vi "DriveModuleControl.vi"(8 "error in":errorcluster, 9 "Actual State":T1={"Speed"=0.0, "Angle"={"VALUE"=0.0, "COS"=1.0, "SIN"=0.0}} {"Angle"."SIN" format="%13.4f"; "Angle"."COS" format="%13.4f"; "Angle"."VALUE" format="%13.4f"}, 10 "Desired State":T1={"Speed"=0.0, "Angle"={"VALUE"=0.0, "COS"=1.0, "SIN"=0.0}} {"Angle"."SIN" format="%13.4f"; "Angle"."COS" format="%13.4f"; "Angle"."VALUE" format="%13.4f"}, 11 "ModualNamePrefix":i32) -> (0 "error out":errorcluster)   [LabVIEW 2023]
uses:
  <vilib>/Rock Robotics/WPI/ThirdParty/JAS_Junk/TrajLib/TypeDef/SWERVE_DRIVE_MODULE_STATE.ctl
  <vilib>/Rock Robotics/WPI/ThirdParty/JAS_Junk/TrajLib/TypeDef/ROTATION2D.ctl
  <vilib>/Rock Robotics/WPI/ThirdParty/JAS_Junk/TrajLib/Rotation2d_Minus.vi
  <vilib>/Rock Robotics/WPI/ThirdParty/JAS_Junk/TrajLib/Rotation2d_GetRadians.vi
  <vilib>/Rock Robotics/WPI/ThirdParty/JAS_Junk/TrajLib/SwerveModuleState_New.vi
  <vilib>/Rock Robotics/WPI/ThirdParty/JAS_Junk/TrajLib/Rotation2d_RotateBy.vi
  <vilib>/Rock Robotics/WPI/ThirdParty/JAS_Junk/TrajLib/Rotation2d_CreateAngle.vi
  <vilib>/Rock Robotics/WPI/ThirdParty/JAS_Junk/TrajLib/SimpleMotorFF_Calculate.vi
  <vilib>/Rock Robotics/WPI/ThirdParty/JAS_Junk/TrajLib/PIDController_AtSetpoint.vi
  <vilib>/Rock Robotics/WPI/ThirdParty/JAS_Junk/TrajLib/PIDController_SetPIDF.vi
  <vilib>/Rock Robotics/WPI/ThirdParty/JAS_Junk/TrajLib/PIDController_SetDerivativeFilter.vi
  <vilib>/Rock Robotics/WPI/ThirdParty/JAS_Junk/TrajLib/PIDController_SetIntegratorRange.vi
  <vilib>/Rock Robotics/WPI/ThirdParty/JAS_Junk/TrajLib/PIDController_SetTolerancePandV.vi
  <vilib>/Rock Robotics/WPI/ThirdParty/JAS_Junk/TrajLib/PIDController_DisableContinousInput.vi
  <vilib>/Rock Robotics/WPI/ThirdParty/JAS_Junk/TrajLib/PIDController_EnableContinousInput.vi
  <vilib>/Rock Robotics/WPI/ThirdParty/JAS_Junk/TrajLib/PIDController_Reset.vi
  <vilib>/Rock Robotics/WPI/ThirdParty/JAS_Junk/TrajLib/PIDController_New.vi
  <vilib>/Rock Robotics/WPI/ThirdParty/JAS_Junk/TrajLib/PIDController_SetOutputLimits.vi
  <vilib>/Rock Robotics/WPI/ThirdParty/JAS_Junk/TrajLib/VI/PIDController_SetIntegratorZone.vi
  <vilib>/Rock Robotics/WPI/ThirdParty/JAS_Junk/TrajLib/SlewRateLimiter_New.vi
  <vilib>/Rock Robotics/WPI/ThirdParty/JAS_Junk/TrajLib/SlewRateLimiter_Reset.vi
  <vilib>/Rock Robotics/WPI/ThirdParty/JAS_Junk/TrajLib/SlewRateLimiter_Calculate.vi
  <vilib>/Rock Robotics/WPI/ThirdParty/JAS_Junk/TrajLib/SlewRateLimiter_SetRate.vi
  <vilib>/Rock Robotics/WPI/ThirdParty/JAS_Junk/TrajLib/Rotation2d_UnaryMinus.vi
  <vilib>/Rock Robotics/WPI/ThirdParty/JAS_Junk/TrajLib/Rotation2d_CreateXY.vi
  <vilib>/Rock Robotics/WPI/ThirdParty/JAS_Junk/TrajLib/PIDController_NewPeriod.vi
  <vilib>/Rock Robotics/WPI/ThirdParty/JAS_Junk/TrajLib/Util_GetTime.vi
  <vilib>/Rock Robotics/WPI/ThirdParty/JAS_Junk/TrajLib/Util_CalcDist.vi
  <vilib>/Rock Robotics/SystemInterfaces/NetworkCommunication/NetComm_UsageReport_report.vi
  <vilib>/Rock Robotics/WPI/ThirdParty/JAS_Junk/TrajLib/VI/Util_GetTime_U32.vi
  DriveGlobal.vi
  <vilib>/Rock Robotics/SystemInterfaces/Utilities/FPGA_UtilitiesRead LocalTime.vi
  <vilib>/Rock Robotics/WPI/ThirdParty/JAS_Junk/TrajLib/VI/Util_GetTime_U64.vi
  <vilib>/Rock Robotics/WPI/ThirdParty/Phoenix-LabVIEW/CANCoder/CTRE_Phoenix_CANcoder_RefNumRegistryGet.vi
  <vilib>/Rock Robotics/WPI/MotorControl/WPI_MotorControlRefNum Registry Get.vi
  <vilib>/Rock Robotics/Network Tables/NT Write Number.vi
  <vilib>/Rock Robotics/WPI/ThirdParty/JAS_Junk/TrajLib/Globals/Util_LibraryGlobals.vi
  <vilib>/Rock Robotics/WPI/ThirdParty/JAS_Junk/TrajLib/PIDController_AdvCalculate_FF_Sp_Pv.vi
  <vilib>/Rock Robotics/WPI/ThirdParty/JAS_Junk/TrajLib/Trajectory_Library.lvlib
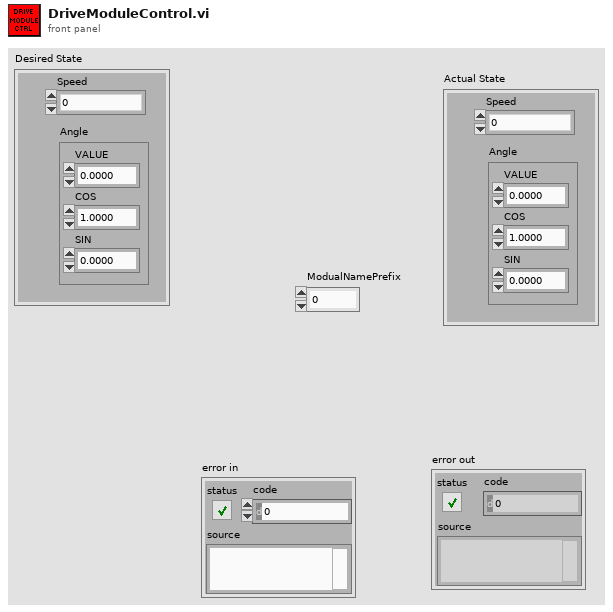
[diagram p1: front panel]
types:
  T1 = typedef "Trajectory_Library.lvlib/SWERVE_DRIVE_MODULE_STATE.ctl" = cluster{"Speed":dbl, "Angle":T2}
  T2 = typedef "Trajectory_Library.lvlib/ROTATION2D.ctl" = cluster{"VALUE":dbl, "COS":dbl, "SIN":dbl}
  T3 = typedef "WPI_MotorControlDeviceRef.ctl" = cluster{"DeviceStatus":errorcluster, "Type":T4, "PWM":cluster{"PWM Channel":T5, "DeadBand":T6}, "CAN":cluster{"Device Number":u8, "SetOutput VI Ref":variant, "GetOutput VI Ref":variant, "Enable VI Ref":variant, "Disable VI Ref":variant, "Data":variant}, "Invert":bool, "DIO PWM":cluster{"PWM \"Enable\" Channel":T5, "DIOChannel":T7, "PWM Rate":dbl}}
  T4 = typedef "WPI_MotorControlType.ctl" = enum16{"PWM", "CAN", "DIO PWM"}
  T5 = typedef "FPGA_DIOPWMChannel.ctl" = enum8{"PWM 0", "PWM 1", "PWM 2", "PWM 3", "PWM 4", "PWM 5", "PWM 6", "PWM 7", "PWM 8", "PWM 9", "PWM MXP 0", "PWM MXP 1", "PWM MXP 2", "PWM MXP 3", "PWM MXP 4", "PWM MXP 5", "PWM MXP 6", "PWM MXP 7", "PWM MXP 8", "PWM MXP 9", "Invalid"}
  T6 = typedef "WPI_PWMDeadband.ctl" = cluster{"Name":string, "maxPositivePwm":i32, "minPositivePwm":i32, "centerPwm":i32, "maxNegativePwm":i32, "minNegativePwm":i32, "angularRange":u16}
  T7 = typedef "FPGA_DIOChannel.ctl" = enum8{"DIO 0", "DIO 1", "DIO 2", "DIO 3", "DIO 4", "DIO 5", "DIO 6", "DIO 7", "DIO 8", "DIO 9", "DIO MXP 0", "DIO MXP 1", "DIO MXP 2", "DIO MXP 3", "DIO MXP 4", "DIO MXP 5", "DIO MXP 6", "DIO MXP 7", "DIO MXP 8", "DIO MXP 9", "DIO MXP 10", "DIO MXP 11", "DIO MXP 12", "DIO MXP 13", "DIO MXP 14", "DIO MXP 15", "SPI Port CS1", "SPI Port CS2", "SPI Port CS3", "SPI Port MISO", "SPI Port MOSI", "Invalid"}
  T8 = typedef "Trajectory_Library.lvlib/SIMPLE_MOTOR_FF.ctl" = cluster{"Ks":dbl, "Kv":dbl, "Ka":dbl, "KnInv":dbl}
  T9 = typedef "Trajectory_Library.lvlib/PID_ADV_LIMITS.ctl" = cluster{"MaxInput":dbl, "MinInput":dbl, "Continuous":bool, "MaxOutput":dbl, "MinOutput":dbl}
  T10 = typedef "Trajectory_Library.lvlib/PID_ADV_TUNING.ctl" = cluster{"Kf":dbl, "Kp":dbl, "Ki":dbl, "Kd":dbl, "MaximumIntegral":dbl, "MinimumIntegral":dbl, "Filter Derivative":bool, "IntegralZone":dbl}
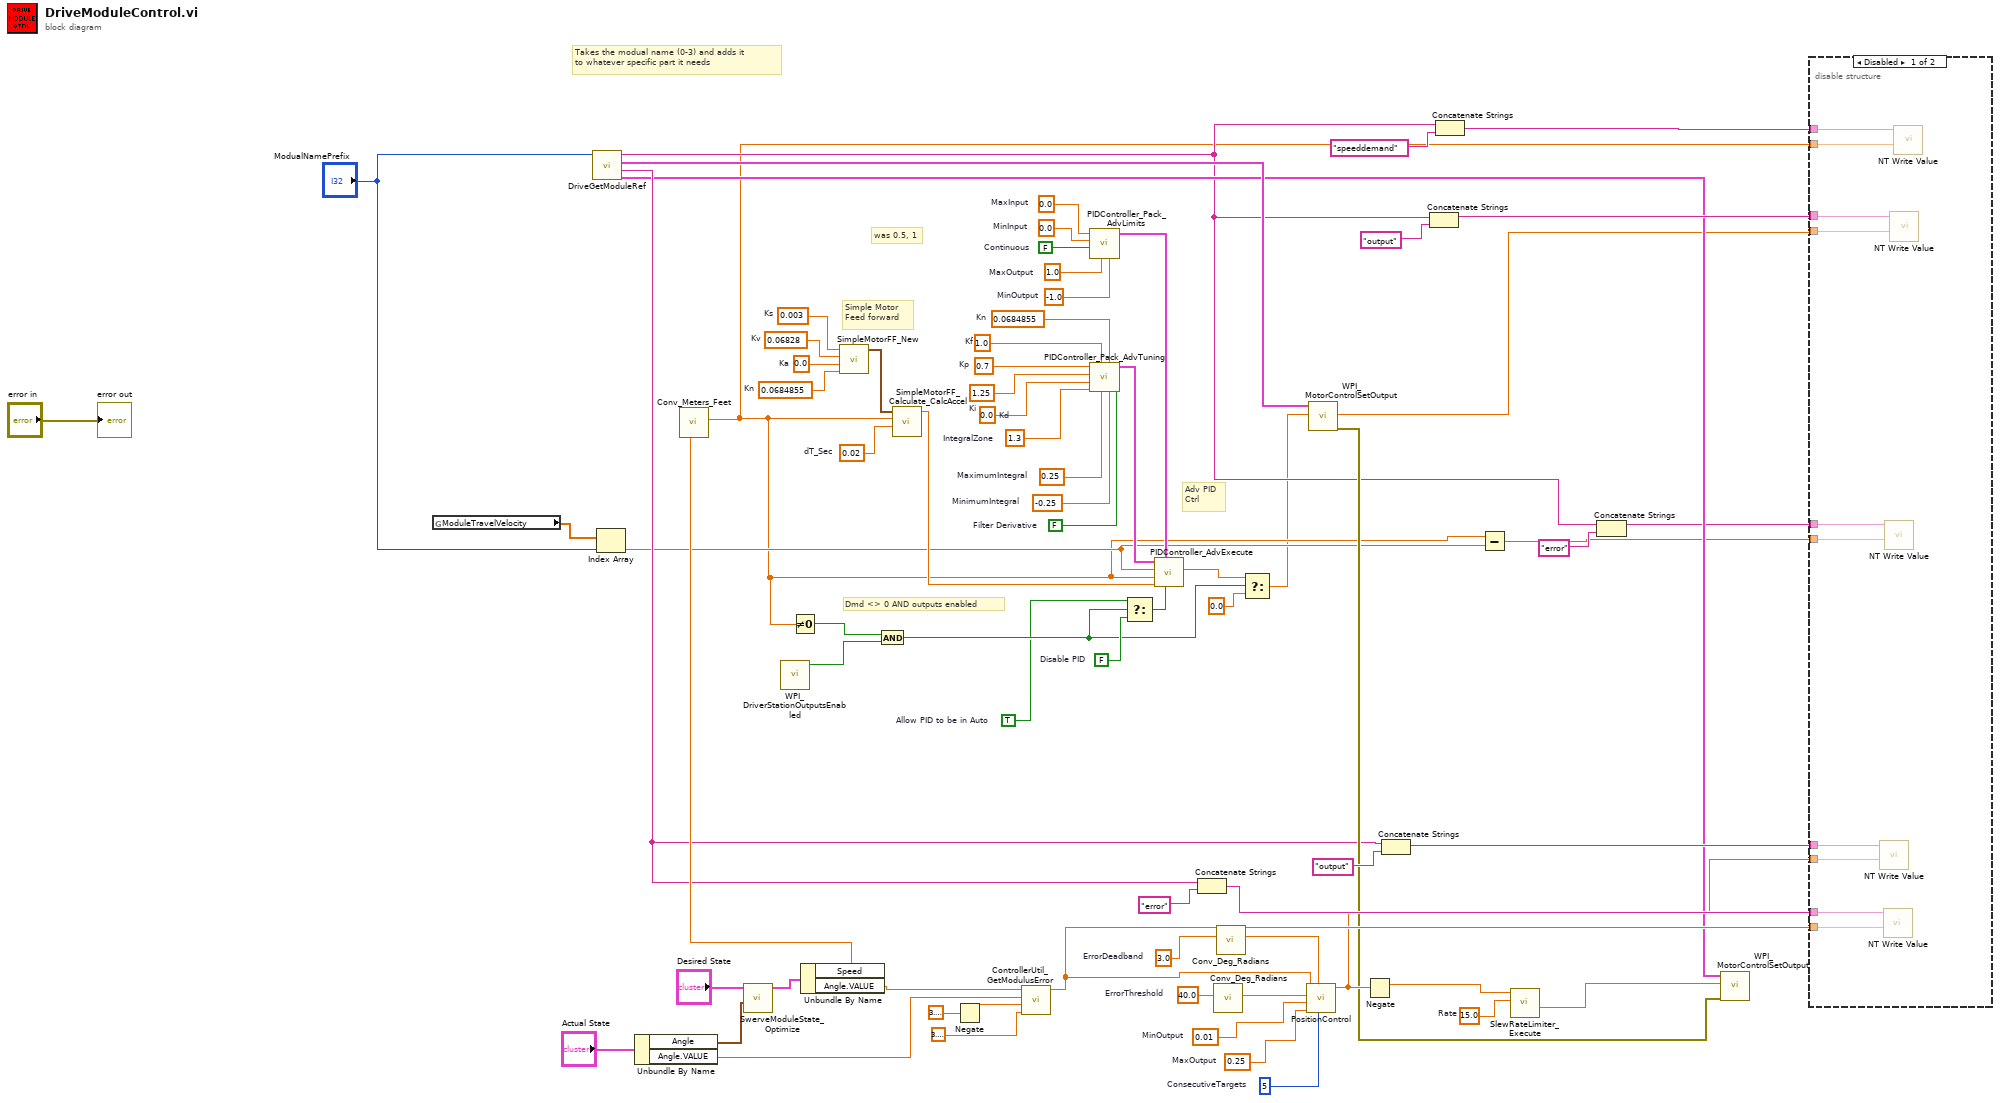
[diagram p0: block diagram]
diagram:
  w1 = 1.3  # IntegralZone
  w4 = 15.0  # Rate
  w5 = TRUE  # Allow PID to be in Auto
  w7 = FALSE  # Disable PID
  w20 = 0.0684855  # Kn
  w37 = 0.7  # Kp
  w36 = 1.25  # Ki
  w35 = 0.0  # Kd
  w34 = 1.0  # Kf
  w33 = 0.25  # MaximumIntegral
  w32 = -0.25  # MinimumIntegral
  w31 = FALSE  # Filter Derivative
  w29 = 0.0  # MinInput
  w28 = FALSE  # Continuous
  w27 = 1.0  # MaxOutput
  w30 = -1.0  # MinOutput
  w26 = 0.0  # MaxInput
  w47 = 0.0684855  # Kn
  w46 = 0.02  # dT_Sec
  w44 = 0.003  # Ks
  w43 = 0.06828  # Kv
  w42 = 0.0  # Ka
  w57 = 5  # ConsecutiveTargets
  w54 = 0.25  # MaxOutput
  w58 = 0.01  # MinOutput
  w51 = 40.0  # ErrorThreshold
  w53 = 3.0  # ErrorDeadband
  # "was 0.5, 1"
  # "Dmd <> 0 AND outputs enabled"
  # "Adv PID\nCtrl"
  # "Simple Motor\nFeed forward"
  # "Takes the modual name (0-3) and adds it \nto whatever specific part it needs"
  n1 = global read "DriveGlobal.vi" "ModuleTravelVelocity"() -> (w22:dbl[])
  n2 = call "DriveGetModuleRef.vi"("ModualNamePrefix"="ModualNamePrefix") -> ("SpinMot"=w38:T3, "SpinStr"=w39:string, "TravMot"=w40:T3, "TravStr"=w15:string)  [unwired: 5 in, 2 out]
  n3 = Index Array(array=w22, index="ModualNamePrefix") -> (element=w19:dbl)
  n4 = Unbundle By Name("Actual State") -> ("Angle"=w65:T2, "Angle.VALUE"=w61:dbl)
  n5 = call <vilib>:"SwerveModuleState_Optimize.vi"("CurrentAngle"=w65, "Desired State"="Desired State") -> ("out SWERVE_DRIVE_MODULE_STATE"=w63:T1)  [unwired: 9 in]
  n6 = call <vilib>:"WPI_DriverStationOutputsEnabled.vi"() -> ("OutputsEnabled?"=w10:bool)  [unwired: 10 in, 1 out]
  n7 = Unbundle By Name(w63) -> ("Speed"=w48:dbl, "Angle.VALUE"=w62:dbl)
  n8 = call <vilib>:"Conv_Meters_Feet.vi"("Meters"=w48) -> ("Feet"=w14:dbl)  [unwired: 10 in]
  n9 = Not Equal To 0?(x=w14) -> (x != 0?=w9:bool)
  n10 = call <vilib>:"SimpleMotorFF_New.vi"("Kn"=w47, "Ka"=w42, "Kv"=w43, "Ks"=w44) -> ("SIMPLE_MOTOR_FF"=w45:T8)  [unwired: 7 in]
  n11 = And(x=w9, y=w10) -> (x .and. y?=w6:bool)
  n12 = call <vilib>:"SimpleMotorFF_Calculate_CalcAccel.vi"("dT_Sec"=w46, "VelSp"=w14, "SIMPLE_MOTOR_FF"=w45) -> ("FeedForward"=w23:dbl)  [unwired: 8 in]
  n13 = Negate(x=3.141592653589793) -> (-x=w64:dbl)
  n14 = call <vilib>:"ControllerUtil_GetModulusError.vi"("Maximum_Input"=3.141592653589793, "Minimum_Input"=w64, "Measurerment(PV)"=w61, "Reference(SP)"=w62) -> ("Error"=w55:dbl)  [unwired: 7 in]
  n15 = call <vilib>:"PIDController_Pack_AdvLimits.vi"("MinOutput"=w30, "MaxOutput"=w27, "Continuous"=w28, "MinInput"=w29, "MaxInput"=w26) -> ("Adv PID Limits"=w24:T9)  [unwired: 6 in]
  n16 = call <vilib>:"PIDController_Pack_AdvTuning.vi"("Filter Derivative"=w31, "MinimumIntegral"=w32, "Kn"=w20, "MaximumIntegral"=w33, "Kf"=w34, "IntegralZone"=w1, "Kd"=w35, "Ki"=w36, "Kp"=w37) -> ("Adv PID Tuning"=w25:T10)  [unwired: 2 in]
  n17 = Select(t=w5, s=w6, f=w7) -> (s? t:f=w8:bool)
  n18 = call <vilib>:"PIDController_AdvExecute.vi"("Auto"=w8, "Adv PID Limits"=w24, "FF-FeedForward"=w23, "SP-SetPoint"=w14, "PV-Measurement"=w19, "Adv PID Tuning"=w25) -> ("CO-ControlOutput"=w12:dbl)  [unwired: 3 in, 2 out]
  n19 = Concatenate Strings(w39, "error" ("refnum name")) -> (w69:string)
  n20 = call <vilib>:"Conv_Deg_Radians.vi"("Degress"=w51) -> ("Radians"=w50:dbl)  [unwired: 10 in]
  n21 = call <vilib>:"Conv_Deg_Radians.vi"("Degress"=w53) -> ("Radians"=w52:dbl)  [unwired: 10 in]
  n22 = Select(t=w12, s=w6, f=0.0 ("t")) -> (s? t:f=w13:dbl)
  n23 = call "PositionControl.vi"("ConsecutiveTargets"=w57, "ErrorDeadband"=w52, "MaxOutput"=w54, "MinOutput"=w58, "ErrorThreshold"=w50, "Error"=w55) -> ("OutputValue"=w49:dbl)  [unwired: 3 in, 2 out]
  n24 = call <vilib>:"WPI_MotorControlSetOutput.vi"("Output"=w13, "MotorControlDevRef"=w40) -> ("error out"=w41:errorcluster)  [unwired: 7 in, 2 out]
  n25 = Negate(x=w49) -> (-x=w3:dbl)
  n26 = Concatenate Strings(w39, "output" ("refnum name")) -> (w56:string)
  n27 = Concatenate Strings(w15, "output" ("refnum name")) -> (w71:string)
  n28 = Concatenate Strings(w15, "speeddemand" ("refnum name")) -> (w73:string)
  n29 = Subtract(x=w14, y=w19) -> (x-y=w16:dbl)
  n30 = call <vilib>:"SlewRateLimiter_Execute.vi"("PositiveRate"=w4, "Input"=w3) -> ("Output"=w2:dbl)  [unwired: 8 in, 1 out]
  n31 = Concatenate Strings(w15, "error" ("refnum name")) -> (w17:string)
  n32 = call <vilib>:"WPI_MotorControlSetOutput.vi"("error in (no error)"=w41, "Output"=w2, "MotorControlDevRef"=w38) -> ()  [unwired: 6 in, 3 out]
  n33 = disable-structure shown="Disabled" {
    disable-tunnel: w73 -> [w85 _]
    disable-tunnel: w71 -> [w84 _]
    disable-tunnel: w69 -> [w83 _]
    disable-tunnel: w56 -> [w82 _]
    disable-tunnel: w55 -> [w81 _]
    disable-tunnel: w49 -> [w80 _]
    disable-tunnel: w17 -> [w79 _]
    disable-tunnel: w16 -> [w78 _]
    disable-tunnel: w14 -> [w77 _]
    disable-tunnel: w13 -> [w76 _]
    frame Disabled {
      n34 = call-poly <vilib>:"NT Write Value.vi"("value"=w80, "name"=w82) -> ()  [unwired: 9 in, 1 out]
      n35 = call-poly <vilib>:"NT Write Value.vi"("value"=w81, "name"=w83) -> ()  [unwired: 9 in, 1 out]
      n36 = call-poly <vilib>:"NT Write Value.vi"("value"=w78, "name"=w79) -> ()  [unwired: 9 in, 1 out]
      n37 = call-poly <vilib>:"NT Write Value.vi"("value"=w76, "name"=w84) -> ()  [unwired: 9 in, 1 out]
      n38 = call-poly <vilib>:"NT Write Value.vi"("value"=w77, "name"=w85) -> ()  [unwired: 9 in, 1 out]
    }
    frame Enabled {
    }
  }
  "error out" <- "error in"
